vi "20210415_00_ATA_FPGA.vi"() -> ()   [LabVIEW 2018]
doc: "This FPGA VI transfers data samples to the host using a stream. The stream is controlled from the host."
uses:
  <vilib>/Platform/TimedLoop/XDataNode/wakeup.ctl
  <vilib>/Platform/TimedLoop/XDataNode/XDNodeRunTimeDep.lvlib
  <vilib>/Platform/TimedLoop/XDataNode/nitl_modes.ctl
  <vilib>/Platform/TimedLoop/XDataNode/timing_clust.ctl
  <vilib>/Platform/TimedLoop/XDataNode/XDataNode.xnode
  <vilib>/eio/EIONode/EIONode.xnode
  <vilib>/rvi/eio/common/nirviEmuTemplateMethod_errors.vi
  <vilib>/rvi/DataTransferAndStorage/Container/XNode/niFpgaContainer.xnode
  <instrlib>/_niInstr/Basic Elements/v1/FPGA/niInstr Basic Elements v1 FPGA.lvlib
  <vilib>/rvi/FXPMathLib/FxpInterpret/XNode/nifxpmath_Interpret.xnode
  <vilib>/rvi/FXPMathLib/FxpMul/XNode/nifxpmath_Multiplier.xnode
  <vilib>/rvi/FXPMathLib/sim/FxpSim.dll
  <vilib>/rvi/FXPMathLib/FxpAdd/XNode/nifxpmath_Add.xnode
  <vilib>/rvi/Analysis/measure/FFT/XNode/niFpgaFFT.xnode
  <instrlib>/_niInstr/Basic Elements/v1/FPGA/Private/Count Up U32.vi
  <vilib>/rvi/Memory/Memory_Emulation/niFpgaMemoryEmulationRefIn.vi
  <vilib>/fxp/LVFixedPointQuantizationPolicyTypeDef.ctl
  <vilib>/rvi/Analysis/measure/FFT/simModelSupport/niFpgaFFTSimDfxp.ctl
  <vilib>/rvi/Analysis/measure/FFT/simModelSupport/niFpgaFFTSimArithmeticProperties.ctl
  <vilib>/rvi/Analysis/measure/FFT/simModelSupport/niFPGA FFT Sim Types.ctl
  <vilib>/rvi/Analysis/measure/FFT/simModelSupport/niFPGA FFT Outside SCTL Sim Properties.ctl
  <vilib>/rvi/Analysis/measure/FFT/simModelSupport/niFpgaFFTSimModelOutsideSCTLCore.vi
  <vilib>/rvi/LocalResourceManager/LocalResourceManager.xnode
  <vilib>/rvi/DataTransferAndStorage/Container/Common/niFpgaContainerGetUniqueNameForEmu.vi
  <vilib>/rvi/DataTransferAndStorage/Container/Common/niFpgaContainerSetEmuInfo.vi
  <vilib>/rvi/eio/common/nirviEmuReportErrorAndStop.vi
  <vilib>/rvi/FIFO/Fifo_Resource/niFpgaFifoEmulationRefIn.vi
  <vilib>/rvi/FIFO/Fifo_Resource/nirvififoEmulationRead.vi
  <vilib>/rvi/interface/RandomDataEmulation/nirviRandomDataFpgaMultiElementTemplate.vi
  <instrlib>/_niInstr/Basic Elements/v1/FPGA/Private/Count Up U16.vi
  FPGA_Controls/FilterStageEnum.ctl
  FPGA_Controls/FPGA_Enable_Clust.ctl
  FPGA_Controls/FPGA_Shift_Enable.ctl
  <instrlib>/_niInstr/Basic Elements/v1/FPGA/Private/Count Up U8.vi
  FPGA_Controls/FPGA_Scale_Clust.ctl
  FPGA_Controls/FPGA_Probe_Clust.ctl
panel:
  out "Write to FIFO 2":bool
  out "Write to FIFO":bool
  in  "EnableFIFO":bool
  out "AI0_Unshifted_Index":u32
  out "AI0_Co_Beac_Q_Index":fxp<+/-,24,1>
  out "AI0_Co_I_Index":fxp<+/-,24,1>
  out "MaxMeas":fxp<+/-,24,1>
  in  "Ramp?":bool
  out "AI1_Over":bool
  out "AI0_Over":bool
  in  "Simulate?":bool
  out "Chan1_Beac_QProbe":T1
  out "Chan1_Beac_IProbe":T1
  out "Chan1_Cal_QProbe":T1
  out "Chan0_Beac_QProbe":T1
  out "Chan0_Beac_IProbe":T1
  out "Chan0_Cal_QProbe":T1
  out "NoiseFloorFFT_LoopCount 2":i32
  out "ReceiverTimed Out 2":bool
  out "SuccessiveIndeces 2":u16[](array[numeric])
  in  "#Avg 2":u16=1
  in  "ScaleMeasurement 2":fxp<+/-,16,1>
  in  "Scale_Step1_2":fxp<+/-,17,17>
  in  "EnableStep1_2":bool
  out "Probe 2_2":fxp<+/-,16,16>
  out "Probe 3_2":fxp<+/-,16,1>
  out "Probe 5_2":fxp<+/-,16,2>
  out "Probe 7_2":fxp<+/-,18,1>
  in  "Scale_NoiseFloor 2":fxp<+/-,30,30>
  out "Probe 21_2":fxp<+/-,24,5>
  out "Probe 22_2":fxp<+/-,54,35>
  out "Probe 23_2":fxp<+/-,54,1>
  out "Probe 24_2":fxp<+/-,16,1>
  in  "Offset 2":fxp<+/-,16,16>
  in  "Scale 2":T2={"Scale_Step4"=1.0, "Scale_Step5"=1.0, "Scale_Step6"=1.0, "Scale_Step7"=1.0}
  in  "Enable 2":T3
  in  "FreqShiftCal 2":fxp<+/-,48,0> format="%#.48g"
  out "Chan1_Cal_IProbe":T1
  in  "FreqShiftBeac 2":fxp<+/-,48,0> format="%#.48g"
  out "NoiseFloorFIFOTimeOut 2":bool
  out "Sends 2":u32
  in  "SampleCountReset 2":u32=125000000
  out "Probe 1_2":i16
  out "Probe Offsetd 2":fxp<+/-,16,16>
  out "Probe Offsetd":fxp<+/-,16,16>
  in  "Sample Clock Commit":bool
  in  "Sample Clock Select":u8
  out "SPI Idle":bool
  out "Configuration Error":bool
  out "Synthesizer Locked":bool
  out "Probe 1":i16
  in  "#Avg":u16=1
  in  "SampleCountReset":u32=125000000
  out "ReceiverTimed Out":bool
  out "Sends":u32
  out "SuccessiveIndeces":u16[](array[numeric])
  out "NoiseFloorFFT_LoopCount":i32
  out "NoiseFloorFIFOTimeOut":bool
  in  "FreqShiftBeac":fxp<+/-,48,0> format="%#.48g"
  out "AI0_Cal_IProbe":T1
  in  "Scale":T2={"Scale_Step4"=1.0, "Scale_Step5"=1.0, "Scale_Step6"=1.0, "Scale_Step7"=1.0}
  in  "Enable":T3
  in  "Offset":fxp<+/-,16,16>
  out "Probe 24":fxp<+/-,16,1>
  out "Probe 23":fxp<+/-,54,1>
  out "Probe 22":fxp<+/-,54,35>
  out "Probe 21":fxp<+/-,24,5>
  in  "Scale_NoiseFloor":fxp<+/-,30,30>
  out "Probe 7":fxp<+/-,18,1>
  out "Probe 5":fxp<+/-,16,2>
  out "Probe 3":fxp<+/-,16,1>
  out "Probe 2":fxp<+/-,16,16>
  in  "EnableStep1":bool
  in  "Scale_Step1":fxp<+/-,17,17>
  in  "ScaleMeasurement":fxp<+/-,16,1>
  in  "FreqShiftCal":fxp<+/-,48,0> format="%#.48g"
  out "IO Module\\Initialization Done":bool
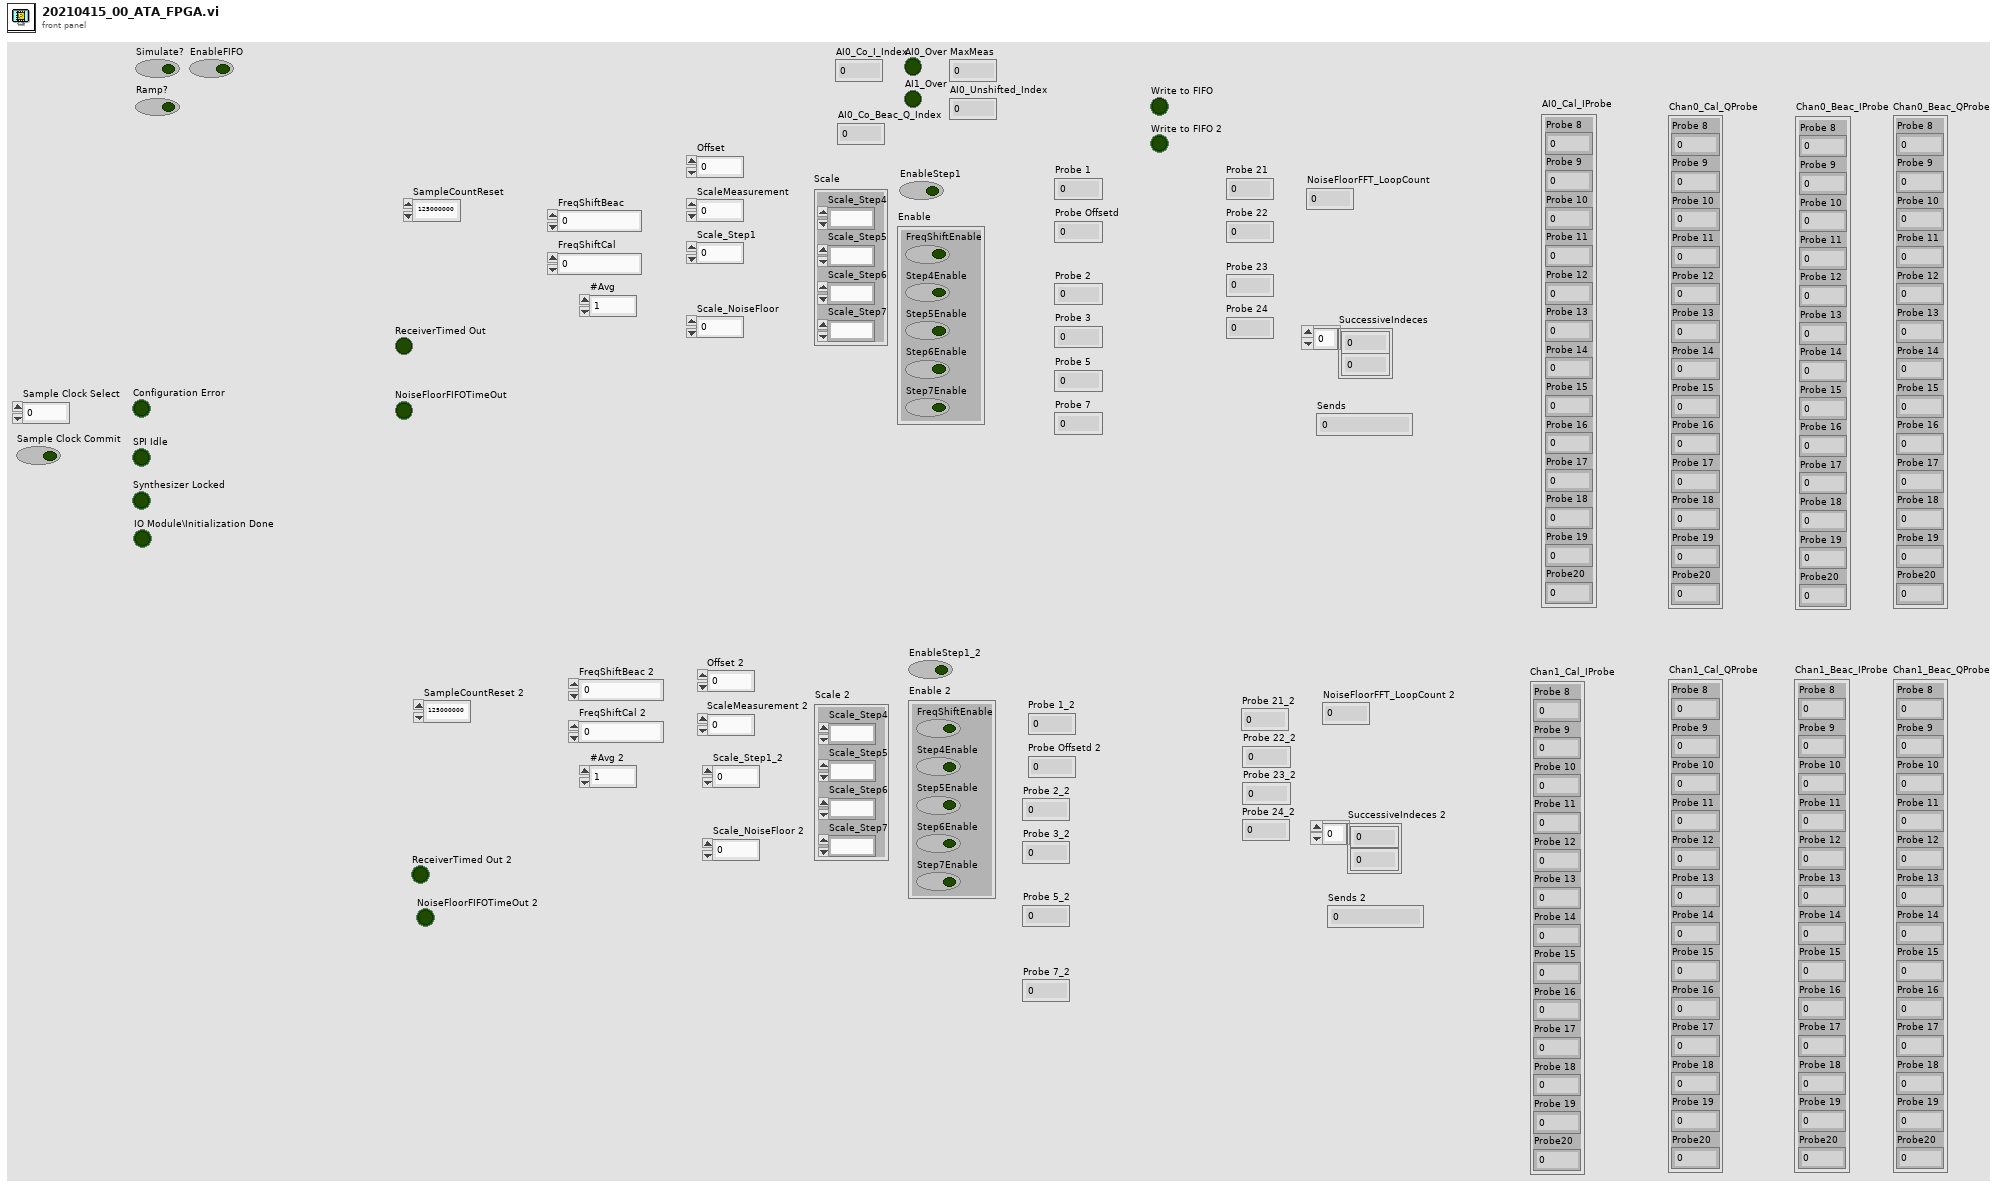
[diagram p1: front panel]
types:
  T1 = typedef "FPGA_Probe_Clust.ctl" = cluster{"Probe 8":fxp<+/-,18,1>, "Probe 9":fxp<+/-,24,1>, "Probe 10":fxp<+/-,24,1>, "Probe 11":fxp<+/-,24,1>, "Probe 12":fxp<+/-,47,24>, "Probe 13":fxp<+/-,24,1>, "Probe 14":fxp<+/-,25,2>, "Probe 15":fxp<+/-,48,25>, "Probe 16":fxp<+/-,24,1>, "Probe 17":fxp<+/-,25,2>, "Probe 18":fxp<+/-,48,25>, "Probe 19":fxp<+/-,24,1>, "Probe20":fxp<+/-,24,1>}
  T2 = typedef "FPGA_Scale_Clust.ctl" = cluster{"Scale_Step4":fxp<+/-,23,23>, "Scale_Step5":fxp<+/-,23,23>, "Scale_Step6":fxp<+/-,23,23>, "Scale_Step7":fxp<+/-,23,23>}
  T3 = typedef "FPGA_Enable_Clust.ctl" = cluster{"FreqShiftEnable":bool, "Step4Enable":bool, "Step5Enable":bool, "Step6Enable":bool, "Step7Enable":bool}
  T4 = typedef "XDNodeRunTimeDep.lvlib/timing_clust.ctl" = cluster{"Expected End [f-1]":u64, "Actual End [f-1]":u64, "Finished Late? [f-1]":bool, "Expected End [i-1]":u64, "Actual End [i-1]":u64, "Finished Late? [i-1]":bool, "Expected Start [i]":u64, "Actual Start [i]":u64, "Expected Start [f]":u64, "Actual Start [f]":u64, "Source Name":string, "Structure Name":string, "Period":i64, "Deadline":i64, "Offset":i64, "Start":i64, "Priority":i32, "Timeout":i32, "Mode":T5, "Wakeup Reason":T6, "Error":errorcluster, "Source Type":string, "Secondary Source Type":string, "Global End Time":u64, "Global Start Time":u64, "Frame Duration":u64, "Iteration Duration":u64, "Assigned CPU":i32, "I/O Scan Engine Mode":u32}
  T5 = typedef "XDNodeRunTimeDep.lvlib/nitl_modes.ctl" = enum32{"No Change", "Process missed periods, maintain original phase", "Discard missed periods, maintain original phase", "Process missed periods, ignore original phase", "Discard missed periods, ignore original phase"}
  T6 = typedef "XDNodeRunTimeDep.lvlib/wakeup.ctl" = enum32{"Normal", "Aborted", "Asynchronous wakeup", "Timing source error", "Timed loop error", "Timeout"}
  T7 = typedef "FPGA_Shift_Enable.ctl" = cluster{"EnableFIFO":bool, "EnableStages":T3}
  T8 = typedef "FilterStageEnum.ctl" = enum16{"Digitiz0", "Digitiz1", "ScaleMeas", "Scale1", "Scale4", "Scale5", "Scale6", "Scale7"}
  T9 = typedef "FPGA_ShiftOutput.ctl" = cluster{"Index":fxp<+/-,24,1>, "output valid":bool, "Data out":fxp<+/-,24,1>, "Probe":T1}
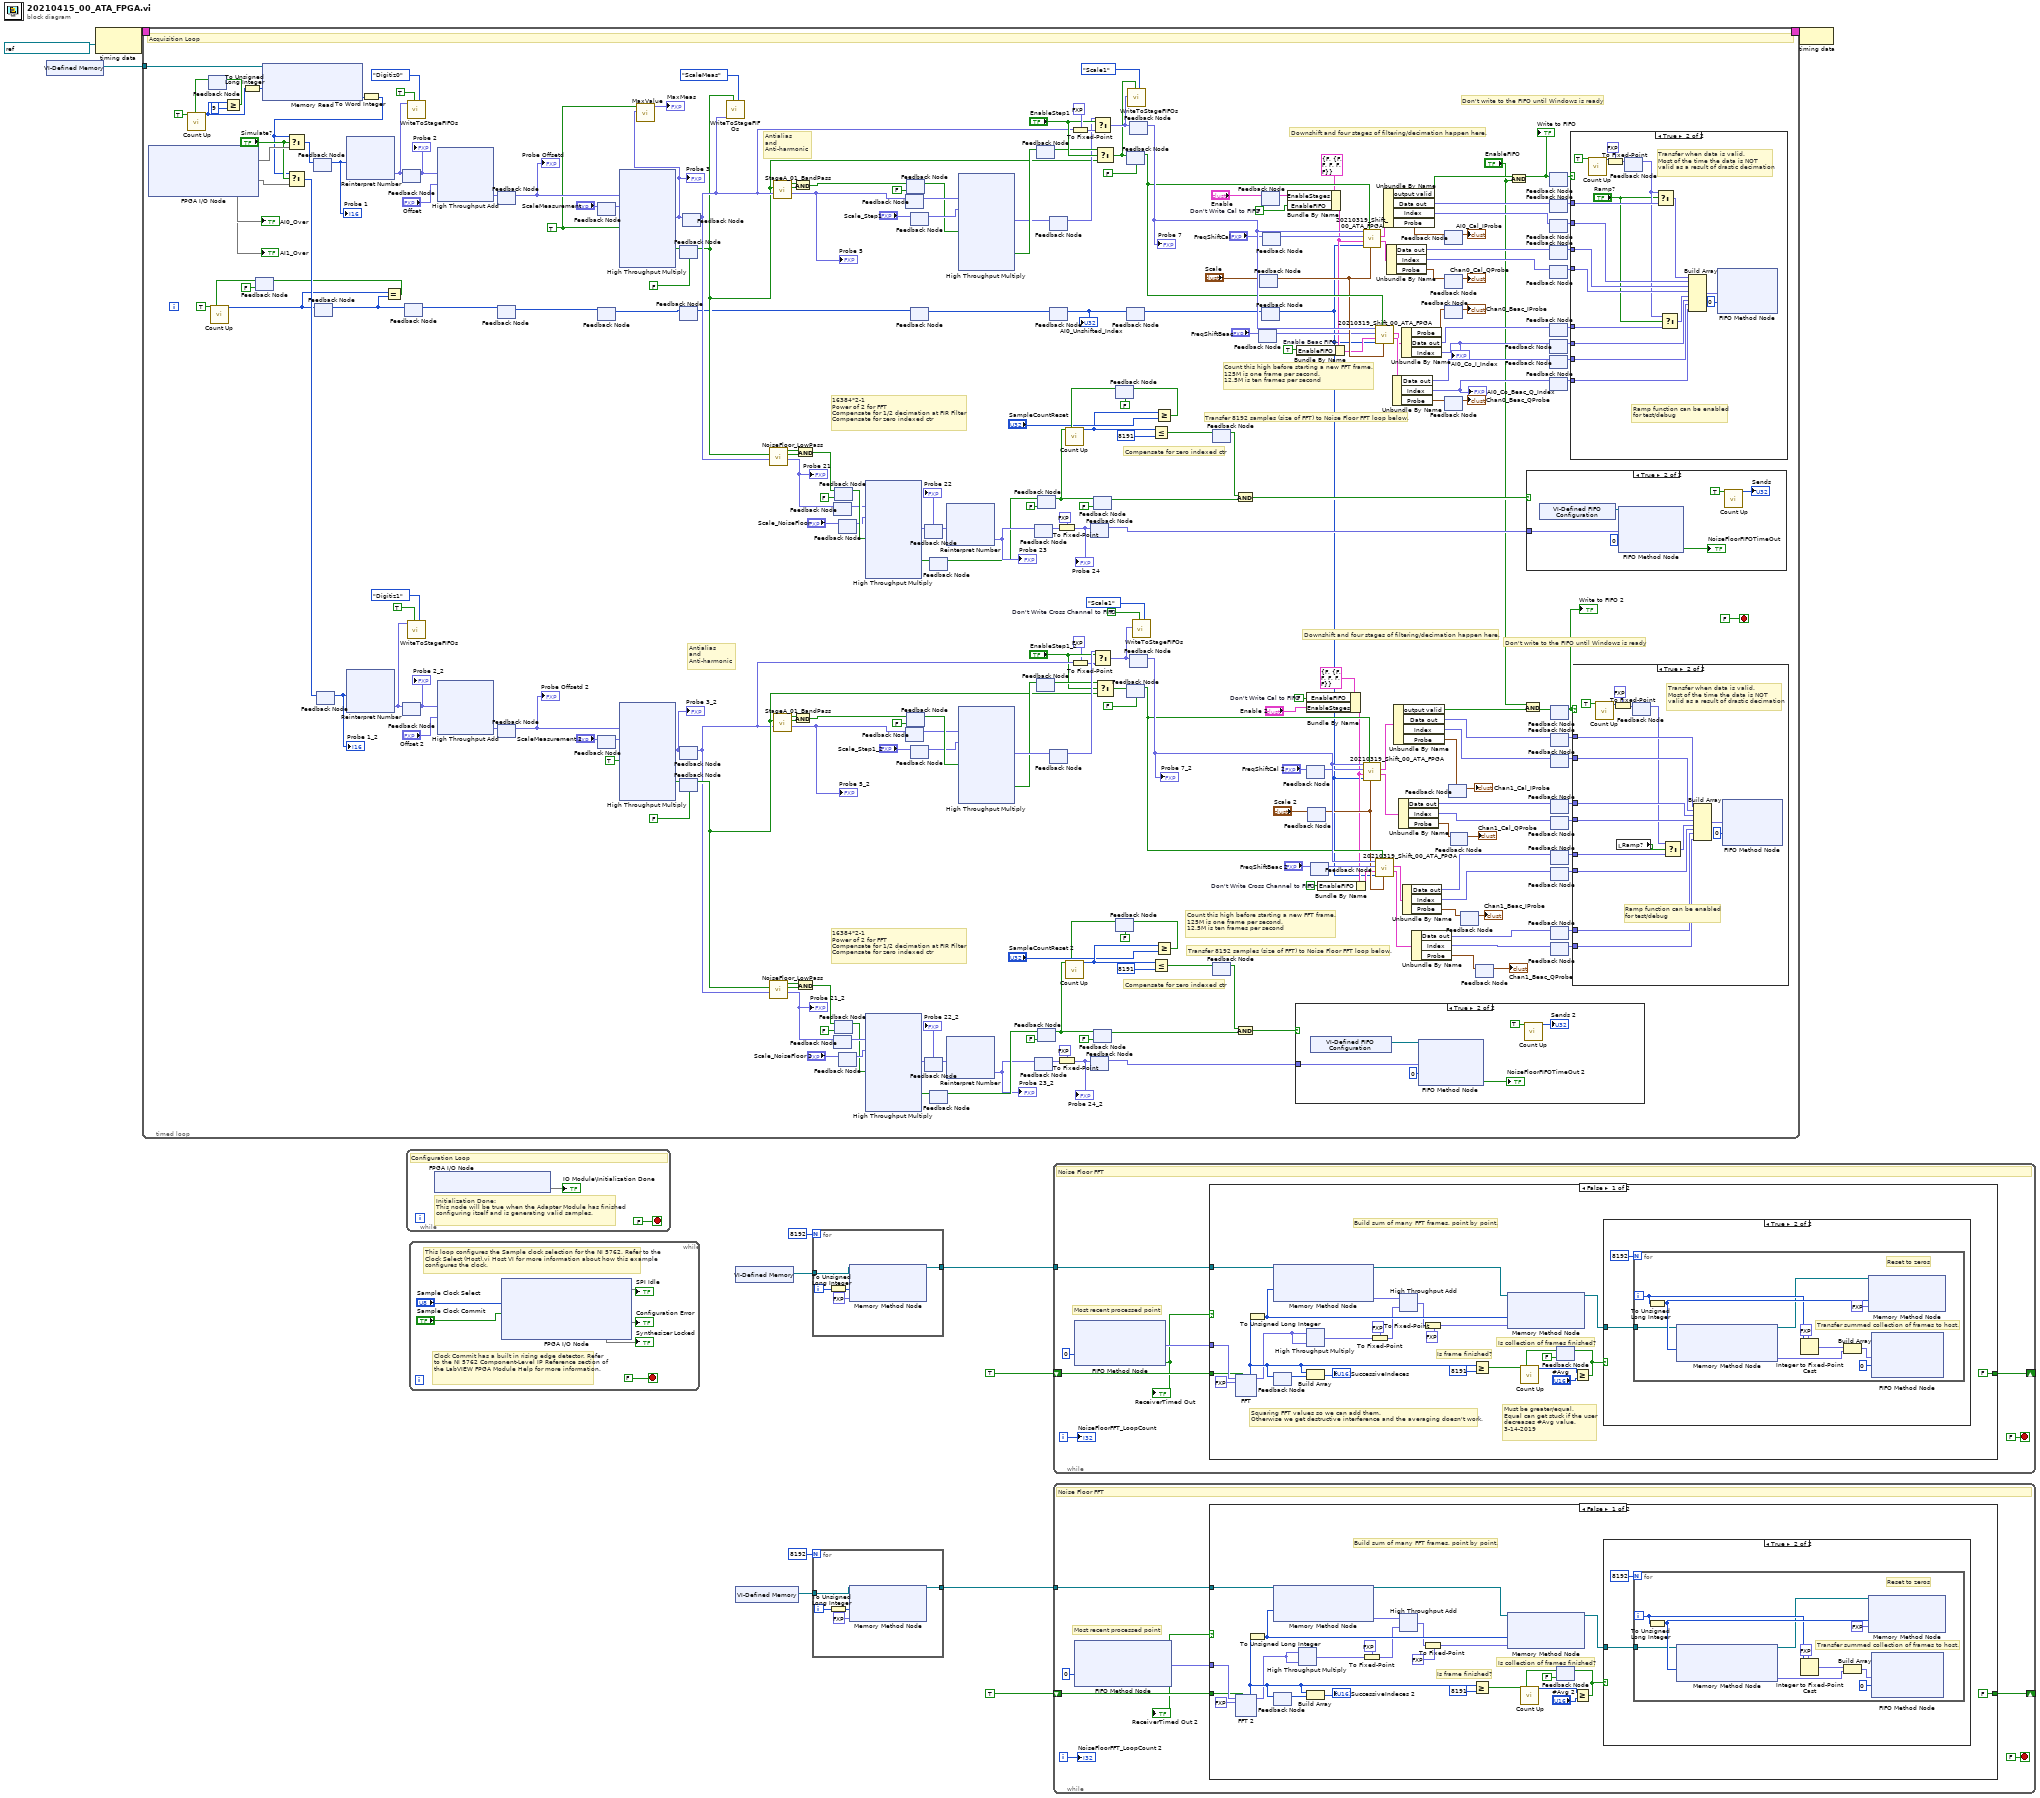
[diagram p0: block diagram]
diagram:
  n1 = xnode "VI-Defined Memory"() -> ("Memory Out"=w1:refnum<k21>)
  n2 = node-c288(refnum<k21> "IO Module\\Data Clock" ("Source Name")) -> (w12:T4)
  n3 = timed-loop {
    timing: w12 -> [_]
    timing-out: [_] -> w11
    tunnel: w1 -> [w111]
    stop <- FALSE stop-if-true
    w59 = FALSE  # Don't Write Cal to FIFO
    w56 = TRUE  # Enable Beac FIFO
    w87 = FALSE  # Don't Write Cross Channel to FIFO
    w45 = FALSE  # Don't Write Cross Channel to FIFO
    w51 = FALSE  # Don't Write Cal to FIFO
    w100 = TRUE ("input valid")
    # "Don't write to the FIFO until Windows is ready"
    # "Don't write to the FIFO until Windows is ready"
    # "Downshift and four stages of filtering/decimation happen here."
    # "Downshift and four stages of filtering/decimation happen here."
    # "Antialias\nand\nAnti-harmonic"
    # "Compensate for zero indexed ctr"
    # "16384*2-1\nPower of 2 for FFT\nCompensate for 1/2 decimation at FIR Filter\nCompensate for zero indexed ctr"
    # "Transfer 8192 samples (size of FFT) to Noise Floor FFT loop below."
    # "Count this high before starting a new FFT frame.\n125M is one frame per second.\n12.5M is ten frames per second"
    # "Antialias\nand\nAnti-harmonic"
    # "Compensate for zero indexed ctr"
    # "16384*2-1\nPower of 2 for FFT\nCompensate for 1/2 decimation at FIR Filter\nCompensate for zero indexed ctr"
    # "Transfer 8192 samples (size of FFT) to Noise Floor FFT loop below."
    # "Count this high before starting a new FFT frame.\n125M is one frame per second.\n12.5M is ten frames per second"
    # "Acquisition Loop"
    n4 = xnode "FPGA I/O Node"() -> ("IO Module\\AI 0 Data"=w110, "IO Module\\AI 0 Over Range"=→"AI0_Over", "IO Module\\AI 1 Data"=w105, "IO Module\\AI 1 Over Range"=→"AI1_Over")  [unwired: 4 in, 4 out]
    n5 = feedback #1() -> (w112:bool)  [unwired: 1 in]
    n6 = call-poly <instrlib>:"Count Up.vi"("increment"=TRUE, "reset"=w112) -> ("count out"=w115:u8)  [unwired: 13 in]
    n7 = Greater Or Equal?(x=w115, y=u8 9) -> (x >= y?=w113:bool)
    n8 = feedback-in #1(w113) -> ()
    n9 = To Unsigned Long Integer(number=w115) -> (unsigned 32bit integer=w117:u32)
    n10 = feedback #2(FALSE) -> (w21:bool)
    n11 = call-poly <instrlib>:"Count Up.vi"("increment"=TRUE, "reset"=w21) -> ("count out"=w19:u32)  [unwired: 13 in]
    n12 = xnode ("Memory Read")("Address"=w117, "Memory In"=w111) -> ("Data"=w108:i8)  [unwired: 1 out]
    n13 = feedback #3() -> (w219:i16)  [unwired: 1 in]
    "Probe 1" <- w219
    n14 = feedback #4() -> (w18:u32)  [unwired: 1 in]
    n15 = feedback-in #4(w19) -> ()
    n16 = feedback #5() -> (w200:i16)  [unwired: 1 in]
    "Probe 1_2" <- w200
    n17 = xnode "Reinterpret Number"("x"=w219) -> ("y"=w91:fxp<+/-,16,16>)
    n18 = xnode "Reinterpret Number"("x"=w200) -> ("y"=w90:fxp<+/-,16,16>)
    n19 = To Word Integer(number=w108) -> (16bit integer=w104:i16)
    n20 = Select(t=w104, s="Simulate?", f=w110) -> (s? t:f=w109:i16)
    n21 = Select(t=w104, s="Simulate?", f=w105) -> (s? t:f=w106:i16)
    n22 = feedback-in #3(w109) -> ()
    n23 = feedback-in #5(w106) -> ()
    n24 = Equal?(x=w19, y=w18) -> (x = y?=w22:bool)
    n25 = feedback-in #2(w22) -> ()
    n26 = feedback #6() -> (w232:fxp<+/-,16,16>)  [unwired: 1 in]
    "Probe 2" <- w232
    n27 = feedback-in #6(w91) -> ()
    n28 = feedback #7() -> (w191:fxp<+/-,16,16>)  [unwired: 1 in]
    "Probe 2_2" <- w191
    n29 = feedback-in #7(w90) -> ()
    n30 = feedback #8() -> (w23:u32)  [unwired: 1 in]
    n31 = feedback-in #8(w18) -> ()
    n32 = call "WriteToStageFIFOs.vi"("Stage"=FilterStageEnum."Digitiz0", "Enable"=TRUE, "Digitiz"=w91) -> ()  [unwired: 9 in]
    n33 = call "WriteToStageFIFOs.vi"("Stage"=FilterStageEnum."Digitiz1", "Enable"=TRUE, "Digitiz"=w90) -> ()  [unwired: 9 in]
    n34 = xnode ("High Throughput Add")("x"=w232, "y"="Offset") -> ("x+y"=w231:fxp<+/-,16,16>)
    n35 = xnode ("High Throughput Add")("x"=w191, "y"="Offset 2") -> ("x+y"=w93:fxp<+/-,16,16>)
    n36 = feedback #9() -> (w101:fxp<+/-,16,16>)  [unwired: 1 in]
    "Probe Offsetd" <- w101
    n37 = feedback-in #9(w231) -> ()
    n38 = feedback #10() -> (w80:u32)  [unwired: 1 in]
    n39 = feedback-in #10(w23) -> ()
    n40 = feedback #11() -> (w92:fxp<+/-,16,16>)  [unwired: 1 in]
    "Probe Offsetd 2" <- w92
    n41 = feedback-in #11(w93) -> ()
    n42 = feedback #12() -> (w260:fxp<+/-,16,1>)  [unwired: 1 in]
    n43 = feedback-in #12("ScaleMeasurement") -> ()
    n44 = feedback #13() -> (w79:u32)  [unwired: 1 in]
    n45 = feedback-in #13(w80) -> ()
    n46 = feedback #14() -> (w161:fxp<+/-,16,1>)  [unwired: 1 in]
    n47 = feedback-in #14("ScaleMeasurement 2") -> ()
    n48 = xnode ("High Throughput Multiply")("x"=w101, "y"=w260, "input valid"=w100) -> ("x*y"=w99:fxp<+/-,16,1>, "output valid"=w234:bool)  [unwired: 1 in, 1 out]
    "Probe 3" <- w99
    n49 = xnode ("High Throughput Multiply")("x"=w92, "y"=w161, "input valid"=TRUE) -> ("x*y"=w158:fxp<+/-,16,1>, "output valid"=w189:bool)  [unwired: 1 in, 1 out]
    "Probe 3_2" <- w158
    n50 = call "MaxValue.vi"("NewValue"=w99, "DataValid"=w100) -> ("Max"=→"MaxMeas":fxp<+/-,24,1>)  [unwired: 9 in]
    n51 = feedback #15(FALSE ("output valid")) -> (w82:bool)
    n52 = feedback-in #15(w234) -> ()
    n53 = feedback #16() -> (w78:u32)  [unwired: 1 in]
    n54 = feedback-in #16(w79) -> ()
    n55 = feedback #17() -> (w203:fxp<+/-,16,1>)  [unwired: 1 in]
    n56 = feedback-in #17(w158) -> ()
    n57 = feedback #18(FALSE ("output valid")) -> (w205:bool)
    n58 = feedback-in #18(w189) -> ()
    n59 = feedback #19() -> (w83:fxp<+/-,16,1>)  [unwired: 1 in]
    n60 = feedback-in #19(w99) -> ()
    n61 = call "WriteToStageFIFOs.vi"("Stage"=FilterStageEnum."ScaleMeas", "Enable"=w82, "ScaleMeas"=w83) -> ()  [unwired: 9 in]
    n62 = call "NoiseFloor_LowPass.vi"("s_axis_data_tdata"=w83, "s_axis_data_tvalid"=w82) -> ("m_axis_data_tdata"=w244:fxp<+/-,24,5>, "m_axis_data_tvalid"=w251:bool, "s_axis_data_tready"=w252:bool)  [unwired: 7 in]
    "Probe 21" <- w244
    n63 = call "NoiseFloor_LowPass.vi"("s_axis_data_tdata"=w203, "s_axis_data_tvalid"=w205) -> ("m_axis_data_tdata"=w179:fxp<+/-,24,5>, "m_axis_data_tvalid"=w172:bool, "s_axis_data_tready"=w171:bool)  [unwired: 7 in]
    "Probe 21_2" <- w179
    n64 = call "StageA_01_BandPass.vi"("s_axis_data_tdata"=w83, "s_axis_data_tvalid"=w82) -> ("m_axis_data_tdata"=w216:fxp<+/-,16,2>, "m_axis_data_tvalid"=w265:bool, "s_axis_data_tready"=w266:bool)  [unwired: 7 in]
    "Probe 5" <- w216
    n65 = call "StageA_01_BandPass.vi"("s_axis_data_tdata"=w203, "s_axis_data_tvalid"=w205) -> ("m_axis_data_tdata"=w204:fxp<+/-,16,2>, "m_axis_data_tvalid"=w155:bool, "s_axis_data_tready"=w154:bool)  [unwired: 7 in]
    "Probe 5_2" <- w204
    n66 = And(x=w266, y=w265) -> (x .and. y?=w217:bool)
    n67 = And(x=w154, y=w155) -> (x .and. y?=w202:bool)
    n68 = And(x=w252, y=w251) -> (x .and. y?=w243:bool)
    n69 = And(x=w171, y=w172) -> (x .and. y?=w180:bool)
    n70 = feedback #20() -> (w245:fxp<+/-,24,5>)  [unwired: 1 in]
    n71 = feedback-in #20(w244) -> ()
    n72 = feedback #21() -> (w178:fxp<+/-,24,5>)  [unwired: 1 in]
    n73 = feedback-in #21(w179) -> ()
    n74 = feedback #22(FALSE ("s_axis_data_tvalid")) -> (w248:bool)
    n75 = feedback-in #22(w243) -> ()
    n76 = feedback #23(FALSE ("s_axis_data_tvalid")) -> (w175:bool)
    n77 = feedback-in #23(w180) -> ()
    n78 = feedback #24() -> (w247:fxp<+/-,30,30>)  [unwired: 1 in]
    n79 = feedback-in #24("Scale_NoiseFloor") -> ()
    n80 = feedback #25() -> (w176:fxp<+/-,30,30>)  [unwired: 1 in]
    n81 = feedback-in #25("Scale_NoiseFloor 2") -> ()
    n82 = xnode ("High Throughput Multiply")("x"=w245, "y"=w247, "input valid"=w248) -> ("x*y"=w240:fxp<+/-,54,35>, "output valid"=w237:bool)  [unwired: 1 in, 1 out]
    "Probe 22" <- w240
    n83 = xnode ("High Throughput Multiply")("x"=w178, "y"=w176, "input valid"=w175) -> ("x*y"=w183:fxp<+/-,54,35>, "output valid"=w186:bool)  [unwired: 1 in, 1 out]
    "Probe 22_2" <- w183
    n84 = feedback #26() -> (w262:fxp<+/-,16,2>)  [unwired: 1 in]
    n85 = feedback-in #26(w216) -> ()
    n86 = feedback #27() -> (w159:fxp<+/-,16,2>)  [unwired: 1 in]
    n87 = feedback-in #27(w204) -> ()
    n88 = feedback #28(FALSE ("s_axis_data_tvalid")) -> (w258:bool)
    n89 = feedback-in #28(w217) -> ()
    n90 = feedback #29(FALSE ("s_axis_data_tvalid")) -> (w163:bool)
    n91 = feedback-in #29(w202) -> ()
    n92 = feedback #30() -> (w259:fxp<+/-,17,17>)  [unwired: 1 in]
    n93 = feedback-in #30("Scale_Step1") -> ()
    n94 = feedback #31() -> (w77:u32)  [unwired: 1 in]
    n95 = feedback-in #31(w78) -> ()
    n96 = feedback #32() -> (w162:fxp<+/-,17,17>)  [unwired: 1 in]
    n97 = feedback-in #32("Scale_Step1_2") -> ()
    n98 = feedback #33() -> (w239:fxp<+/-,54,35>)  [unwired: 1 in]
    n99 = feedback-in #33(w240) -> ()
    n100 = feedback #34() -> (w184:fxp<+/-,54,35>)  [unwired: 1 in]
    n101 = feedback-in #34(w183) -> ()
    n102 = feedback #35() -> (w236:bool)  [unwired: 1 in]
    n103 = feedback-in #35(w237) -> ()
    n104 = feedback #36() -> (w187:bool)  [unwired: 1 in]
    n105 = feedback-in #36(w186) -> ()
    n106 = xnode "Reinterpret Number"("x"=w239) -> ("y"=w238:fxp<+/-,54,1>)
    "Probe 23" <- w238
    n107 = xnode "Reinterpret Number"("x"=w184) -> ("y"=w185:fxp<+/-,54,1>)
    "Probe 23_2" <- w185
    n108 = xnode ("High Throughput Multiply")("x"=w262, "y"=w259, "input valid"=w258) -> ("x*y"=w213:fxp<+/-,18,1>, "output valid"=w215:bool)  [unwired: 1 in, 1 out]
    n109 = xnode ("High Throughput Multiply")("x"=w159, "y"=w162, "input valid"=w163) -> ("x*y"=w208:fxp<+/-,18,1>, "output valid"=w206:bool)  [unwired: 1 in, 1 out]
    n110 = feedback #37() -> (w241:fxp<+/-,54,1>)  [unwired: 1 in]
    n111 = feedback-in #37(w238) -> ()
    n112 = feedback #38() -> (w182:fxp<+/-,54,1>)  [unwired: 1 in]
    n113 = feedback-in #38(w185) -> ()
    n114 = feedback #39() -> (w214:bool)  [unwired: 1 in]
    n115 = feedback-in #39(w215) -> ()
    n116 = feedback #40() -> (w207:bool)  [unwired: 1 in]
    n117 = feedback-in #40(w206) -> ()
    n118 = feedback #41(FALSE ("output valid")) -> (w230:bool)
    n119 = feedback-in #41(w236) -> ()
    n120 = feedback #42(FALSE ("output valid")) -> (w192:bool)
    n121 = feedback-in #42(w187) -> ()
    n122 = feedback #43() -> (w212:fxp<+/-,18,1>)  [unwired: 1 in]
    n123 = feedback-in #43(w213) -> ()
    n124 = feedback #44() -> (w76:u32)  [unwired: 1 in]
    "AI0_Unshifted_Index" <- w76
    n125 = feedback-in #44(w77) -> ()
    n126 = feedback #45() -> (w209:fxp<+/-,18,1>)  [unwired: 1 in]
    n127 = feedback-in #45(w208) -> ()
    n128 = To Fixed-Point(fixed-point type=fxp<+/-,16,1> 0.0, number=w241) -> (fixed-point=w220:fxp<+/-,16,1>)
    "Probe 24" <- w220
    n129 = To Fixed-Point(fixed-point type=fxp<+/-,16,1> 0.0, number=w182) -> (fixed-point=w199:fxp<+/-,16,1>)
    "Probe 24_2" <- w199
    n130 = To Fixed-Point(fixed-point type=fxp<+/-,18,1> 0.0, number=w83) -> (fixed-point=w256:fxp<+/-,18,1>)
    n131 = To Fixed-Point(fixed-point type=fxp<+/-,18,1> 0.0, number=w203) -> (fixed-point=w166:fxp<+/-,18,1>)
    n132 = feedback #46() -> (w221:fxp<+/-,16,1>)  [unwired: 1 in]
    n133 = feedback-in #46(w220) -> ()
    n134 = feedback #47() -> (w198:fxp<+/-,16,1>)  [unwired: 1 in]
    n135 = feedback-in #47(w199) -> ()
    n136 = feedback #48(FALSE ("output valid")) -> (w228:bool)
    n137 = feedback-in #48(w230) -> ()
    n138 = feedback #49(FALSE ("output valid")) -> (w194:bool)
    n139 = feedback-in #49(w192) -> ()
    n140 = Select(t=w212, s="EnableStep1", f=w256) -> (s? t:f=w95:fxp<+/-,18,1>)
    n141 = Select(t=w209, s="EnableStep1_2", f=w166) -> (s? t:f=w88:fxp<+/-,18,1>)
    n142 = Select(t=w214, s="EnableStep1", f=w82) -> (s? t:f=w81:bool)
    n143 = Select(t=w207, s="EnableStep1_2", f=w205) -> (s? t:f=w164:bool)
    n144 = feedback #50(FALSE ("reset")) -> (w271:bool)
    n145 = call-poly <instrlib>:"Count Up.vi"("increment"=w230, "reset"=w271) -> ("count out"=w264:u32)  [unwired: 13 in]
    n146 = feedback #51(FALSE ("reset")) -> (w149:bool)
    n147 = call-poly <instrlib>:"Count Up.vi"("increment"=w192, "reset"=w149) -> ("count out"=w156:u32)  [unwired: 13 in]
    n148 = feedback #52(FALSE ("s_axis_data_tvalid")) -> (w147:bool)
    n149 = feedback-in #52(w81) -> ()
    n150 = feedback #53() -> (w75:u32)  [unwired: 1 in]
    n151 = feedback-in #53(w76) -> ()
    n152 = feedback #54(FALSE ("s_axis_data_tvalid")) -> (w141:bool)
    n153 = feedback-in #54(w164) -> ()
    n154 = call "WriteToStageFIFOs.vi"("Stage"=FilterStageEnum."Scale1", "Enable"=w81, "Scale1"=w95) -> ()  [unwired: 9 in]
    n155 = feedback #55() -> (w211:fxp<+/-,18,1>)  [unwired: 1 in]
    "Probe 7" <- w211
    n156 = feedback-in #55(w95) -> ()
    n157 = feedback #56() -> (w210:fxp<+/-,18,1>)  [unwired: 1 in]
    "Probe 7_2" <- w210
    n158 = feedback-in #56(w88) -> ()
    n159 = call "WriteToStageFIFOs.vi"("Stage"=FilterStageEnum."Scale1", "Enable"=w87, "Scale1"=w88) -> ()  [unwired: 9 in]
    n160 = Less Or Equal?(x=w264, y=u32 8191) -> (x <= y?=w272:bool)
    n161 = Less Or Equal?(x=w156, y=u32 8191) -> (x <= y?=w148:bool)
    n162 = Greater Or Equal?(x=w264, y="SampleCountReset") -> (x >= y?=w268:bool)
    n163 = feedback-in #50(w268) -> ()
    n164 = Greater Or Equal?(x=w156, y="SampleCountReset 2") -> (x >= y?=w152:bool)
    n165 = feedback-in #51(w152) -> ()
    n166 = feedback #57() -> (w229:bool)  [unwired: 1 in]
    n167 = feedback-in #57(w272) -> ()
    n168 = feedback #58() -> (w193:bool)  [unwired: 1 in]
    n169 = feedback-in #58(w148) -> ()
    n170 = And(x=w229, y=w228) -> (x .and. y?=w227:bool)
    n171 = And(x=w193, y=w194) -> (x .and. y?=w195:bool)
    n172 = feedback #59() -> (w130:fxp<+/-,48,0>)  [unwired: 1 in]
    n173 = feedback-in #59("FreqShiftBeac") -> ()
    n174 = feedback #60() -> (w132:T2)  [unwired: 1 in]
    n175 = feedback-in #60("Scale") -> ()
    n176 = feedback #61() -> (w60:T3)  [unwired: 1 in]
    n177 = feedback-in #61("Enable") -> ()
    n178 = feedback #62() -> (w17:u32)  [unwired: 1 in]
    n179 = feedback-in #62(w75) -> ()
    n180 = feedback #63() -> (w128:fxp<+/-,48,0>)  [unwired: 1 in]
    n181 = feedback-in #63("FreqShiftCal") -> ()
    n182 = Bundle By Name(cluster=T7 {"EnableFIFO"=FALSE, "EnableStages"={"FreqShiftEnable"=FALSE, "Step4Enable"=FALSE, "Step5Enable"=FALSE, "Step6Enable"=FALSE, "Step7Enable"=FALSE}}, "EnableStages"=w60, "EnableFIFO"=w59) -> (w58:T7)
    n183 = case shown="True" w195 {
      tunnel: w198 -> [_ w278]
      frame False {
      }
      frame True {
        n184 = xnode "VI-Defined FIFO Configuration"() -> ("FIFO Out"=w273:refnum<k21>)
        n185 = xnode ("FIFO Method Node")("Element"=w278, "Timeout"=0, "FIFO In"=w273) -> ("Timed Out?"=→"NoiseFloorFIFOTimeOut 2":bool)  [unwired: 1 out]
        n186 = call-poly <instrlib>:"Count Up.vi"("increment"=TRUE) -> ("count out"=→"Sends 2":u32)  [unwired: 14 in]
      }
    }
    n187 = Bundle By Name(cluster=w58, "EnableFIFO"=w56) -> (w57:T7)
    n188 = Bundle By Name(cluster=T7 {"EnableFIFO"=FALSE, "EnableStages"={"FreqShiftEnable"=FALSE, "Step4Enable"=FALSE, "Step5Enable"=FALSE, "Step6Enable"=FALSE, "Step7Enable"=FALSE}}, "EnableFIFO"=w51, "EnableStages"="Enable 2") -> (w43:T7)
    n189 = feedback #64() -> (w126:fxp<+/-,48,0>)  [unwired: 1 in]
    n190 = feedback-in #64("FreqShiftCal 2") -> ()
    n191 = feedback #65() -> (w118:T2)  [unwired: 1 in]
    n192 = feedback-in #65("Scale 2") -> ()
    n193 = feedback #66() -> (w124:fxp<+/-,48,0>)  [unwired: 1 in]
    n194 = feedback-in #66("FreqShiftBeac 2") -> ()
    n195 = Bundle By Name(cluster=w43, "EnableFIFO"=w45) -> (w44:T7)
    n196 = call "20210319_Shift_00_ATA_FPGA.vi"("Scale"=w132, "Input valid"=w147, "Index"=w17, "Enable"=w58, "frequency shift"=w128, "Data in"=w211) -> ("Q Shift Output"=w146:T9, "I Shift Output"=w140:T9)  [unwired: 4 in]
    n197 = call "20210319_Shift_00_ATA_FPGA.vi"("Scale"=w118, "Input valid"=w141, "Index"=w17, "Enable"=w43, "frequency shift"=w126, "Data in"=w210) -> ("Q Shift Output"=w42:T9, "I Shift Output"=w50:T9)  [unwired: 4 in]
    n198 = call "20210319_Shift_00_ATA_FPGA.vi"("Scale"=w132, "Input valid"=w147, "Index"=w17, "Enable"=w57, "frequency shift"=w130, "Data in"=w211) -> ("Q Shift Output"=w225:T9, "I Shift Output"=w137:T9)  [unwired: 4 in]
    n199 = call "20210319_Shift_00_ATA_FPGA.vi"("Scale"=w118, "Input valid"=w141, "Index"=w17, "Enable"=w44, "frequency shift"=w124, "Data in"=w210) -> ("Q Shift Output"=w31:T9, "I Shift Output"=w35:T9)  [unwired: 4 in]
    n200 = Unbundle By Name(w140) -> ("output valid"=w72:bool, "Data out"=w65:fxp<+/-,24,1>, "Index"=w67:fxp<+/-,24,1>, "Probe"=w74:T1)
    n201 = Unbundle By Name(w146) -> ("Data out"=w63:fxp<+/-,24,1>, "Index"=w73:fxp<+/-,24,1>, "Probe"=w53:T1)
    n202 = Unbundle By Name(w225) -> ("Data out"=w70:fxp<+/-,24,1>, "Index"=w25:fxp<+/-,24,1>, "Probe"=w69:T1)
    "AI0_Co_Beac_Q_Index" <- w25
    n203 = Unbundle By Name(w50) -> ("output valid"=w49:bool, "Data out"=w48:fxp<+/-,24,1>, "Index"=w47:fxp<+/-,24,1>, "Probe"=w41:T1)
    n204 = Unbundle By Name(w42) -> ("Data out"=w38:fxp<+/-,24,1>, "Index"=w37:fxp<+/-,24,1>, "Probe"=w40:T1)
    n205 = Unbundle By Name(w137) -> ("Probe"=w71:T1, "Data out"=w68:fxp<+/-,24,1>, "Index"=w55:fxp<+/-,24,1>)
    "AI0_Co_I_Index" <- w55
    n206 = Unbundle By Name(w35) -> ("Data out"=w32:fxp<+/-,24,1>, "Index"=w33:fxp<+/-,24,1>, "Probe"=w34:T1)
    n207 = Unbundle By Name(w31) -> ("Data out"=w29:fxp<+/-,24,1>, "Index"=w27:fxp<+/-,24,1>, "Probe"=w30:T1)
    n208 = feedback #67() -> (→"AI0_Cal_IProbe":T1)  [unwired: 1 in]
    n209 = feedback-in #67(w74) -> ()
    n210 = feedback #68() -> (→"Chan0_Cal_QProbe":T1)  [unwired: 1 in]
    n211 = feedback-in #68(w53) -> ()
    n212 = feedback #69() -> (→"Chan0_Beac_IProbe":T1)  [unwired: 1 in]
    n213 = feedback-in #69(w71) -> ()
    n214 = feedback #70() -> (→"Chan0_Beac_QProbe":T1)  [unwired: 1 in]
    n215 = feedback-in #70(w69) -> ()
    n216 = feedback #71() -> (→"Chan1_Cal_IProbe":T1)  [unwired: 1 in]
    n217 = feedback-in #71(w41) -> ()
    n218 = feedback #72() -> (→"Chan1_Cal_QProbe":T1)  [unwired: 1 in]
    n219 = feedback-in #72(w40) -> ()
    n220 = feedback #73() -> (→"Chan1_Beac_IProbe":T1)  [unwired: 1 in]
    n221 = feedback-in #73(w34) -> ()
    n222 = feedback #74() -> (→"Chan1_Beac_QProbe":T1)  [unwired: 1 in]
    n223 = feedback-in #74(w30) -> ()
    n224 = And(x=w72, y="EnableFIFO") -> (x .and. y?=w16:bool)
    "Write to FIFO" <- w16
    n225 = And(x="EnableFIFO", y=w49) -> (x .and. y?=w15:bool)
    n226 = case shown="True" w227 {
      tunnel: w221 -> [_ w301]
      frame False {
      }
      frame True {
        n227 = xnode "VI-Defined FIFO Configuration"() -> ("FIFO Out"=w296:refnum<k21>)
        n228 = xnode ("FIFO Method Node")("Element"=w301, "Timeout"=0, "FIFO In"=w296) -> ("Timed Out?"=→"NoiseFloorFIFOTimeOut":bool)  [unwired: 1 out]
        n229 = call-poly <instrlib>:"Count Up.vi"("increment"=TRUE) -> ("count out"=→"Sends":u32)  [unwired: 14 in]
      }
    }
    n230 = feedback #75() -> (w222:bool)  [unwired: 1 in]
    n231 = feedback-in #75(w16) -> ()
    n232 = feedback #76() -> (w223:fxp<+/-,24,1>)  [unwired: 1 in]
    n233 = feedback-in #76(w65) -> ()
    n234 = feedback #77() -> (w66:fxp<+/-,24,1>)  [unwired: 1 in]
    n235 = feedback-in #77(w67) -> ()
    n236 = feedback #78() -> (w62:fxp<+/-,24,1>)  [unwired: 1 in]
    n237 = feedback-in #78(w63) -> ()
    n238 = feedback #79() -> (w144:fxp<+/-,24,1>)  [unwired: 1 in]
    n239 = feedback-in #79(w73) -> ()
    n240 = feedback #80() -> (w145:fxp<+/-,24,1>)  [unwired: 1 in]
    n241 = feedback-in #80(w68) -> ()
    n242 = feedback #81() -> (w54:fxp<+/-,24,1>)  [unwired: 1 in]
    n243 = feedback-in #81(w55) -> ()
    n244 = feedback #82() -> (w224:fxp<+/-,24,1>)  [unwired: 1 in]
    n245 = feedback-in #82(w70) -> ()
    n246 = feedback #83() -> (w64:fxp<+/-,24,1>)  [unwired: 1 in]
    n247 = feedback-in #83(w25) -> ()
    n248 = feedback #84() -> (w13:bool)  [unwired: 1 in]
    "Write to FIFO 2" <- w13
    n249 = feedback-in #84(w15) -> ()
    n250 = feedback #85() -> (w197:fxp<+/-,24,1>)  [unwired: 1 in]
    n251 = feedback-in #85(w48) -> ()
    n252 = feedback #86() -> (w39:fxp<+/-,24,1>)  [unwired: 1 in]
    n253 = feedback-in #86(w47) -> ()
    n254 = feedback #87() -> (w142:fxp<+/-,24,1>)  [unwired: 1 in]
    n255 = feedback-in #87(w38) -> ()
    n256 = feedback #88() -> (w36:fxp<+/-,24,1>)  [unwired: 1 in]
    n257 = feedback-in #88(w37) -> ()
    n258 = feedback #89() -> (w143:fxp<+/-,24,1>)  [unwired: 1 in]
    n259 = feedback-in #89(w32) -> ()
    n260 = feedback #90() -> (w196:fxp<+/-,24,1>)  [unwired: 1 in]
    n261 = feedback-in #90(w33) -> ()
    n262 = feedback #91() -> (w28:fxp<+/-,24,1>)  [unwired: 1 in]
    n263 = feedback-in #91(w29) -> ()
    n264 = feedback #92() -> (w26:fxp<+/-,24,1>)  [unwired: 1 in]
    n265 = feedback-in #92(w27) -> ()
    n266 = case shown="True" w222 {
      tunnel: w223 -> [_ w315]
      tunnel: w224 -> [_ w304]
      tunnel: w145 -> [_ w302]
      tunnel: w144 -> [_ w310]
      tunnel: w66 -> [_ w313]
      tunnel: w62 -> [_ w311]
      tunnel: w64 -> [_ w312]
      tunnel: w54 -> [_ w309]
      frame False {
        # "Ready last time?"
      }
      frame True {
        # "Ramp function can be enabled\nfor test/debug"
        # "Transfer when data is valid.\nMost of the time the data is NOT\nvalid as a result of drastic decimation"
        n267 = call-poly <instrlib>:"Count Up.vi"("increment"=TRUE) -> ("count out"=w317:u32)  [unwired: 14 in]
        n268 = To Fixed-Point(fixed-point type=fxp<+/-,24,1> 0.0, number=w317) -> (fixed-point=w316:fxp<+/-,24,1>)
        n269 = feedback-in #93(w316) -> ()
        n270 = feedback #93() -> (w306:fxp<+/-,24,1>)  [unwired: 1 in]
        n271 = Select(t=w306, s="Ramp?", f=w315) -> (s? t:f=w314:fxp<+/-,24,1>)
        n272 = Select(t=w306, s="Ramp?", f=w302) -> (s? t:f=w303:fxp<+/-,24,1>)
        n273 = Build Array(w314, w313, w311, w310, w303, w309, w304, w312) -> (w308:fxp<+/-,24,1>[])
        n274 = xnode ("FIFO Method Node")("Element"=w308, "Timeout"=0) -> ()  [unwired: 1 in, 2 out]
      }
    }
    n275 = case shown="True" w13 {
      tunnel: w197 -> [_ w294]
      tunnel: w196 -> [_ w290]
      tunnel: w143 -> [_ w282]
      tunnel: w142 -> [_ w292]
      tunnel: w39 -> [_ w293]
      tunnel: w36 -> [_ w291]
      tunnel: w28 -> [_ w289]
      tunnel: w26 -> [_ w288]
      frame False {
      }
      frame True {
        # "Ramp function can be enabled\nfor test/debug"
        # "Transfer when data is valid.\nMost of the time the data is NOT\nvalid as a result of drastic decimation"
        n276 = call-poly <instrlib>:"Count Up.vi"("increment"=TRUE) -> ("count out"=w285:u32)  [unwired: 14 in]
        n277 = To Fixed-Point(fixed-point type=fxp<+/-,24,1> 0.0, number=w285) -> (fixed-point=w284:fxp<+/-,24,1>)
        n278 = local read "Ramp?"() -> (w280:bool)
        n279 = feedback #94() -> (w283:fxp<+/-,24,1>)  [unwired: 1 in]
        n280 = feedback-in #94(w284) -> ()
        n281 = Select(t=w283, s=w280, f=w282) -> (s? t:f=w281:fxp<+/-,24,1>)
        n282 = Build Array(w294, w293, w292, w291, w281, w290, w289, w288) -> (w295:fxp<+/-,24,1>[])
        n283 = xnode ("FIFO Method Node")("Element"=w295, "Timeout"=0) -> ()  [unwired: 1 in, 2 out]
      }
    }
  }
  n284 = while {
    stop <- FALSE stop-if-true
    # "Initialization Done:\nThis node will be true when the Adapter Module has finished configuring itself and is generating valid samples."
    # "Configuration Loop"
    n285 = xnode "FPGA I/O Node"() -> ("IO Module\\Initialization Done"=→"IO Module\\Initialization Done")  [unwired: 1 in, 1 out]
  }
  n286 = while {
    stop <- FALSE stop-if-true
    # "Clock Commit has a built in rising edge detector. Refer to the NI 5762 Component-Level IP Reference section of the LabVIEW FPGA Module Help for more information."
    # "This loop configures the Sample clock selection for the NI 5762. Refer to the Clock Select (Host).vi Host VI for more information about how this example configures the clock."
    n287 = xnode "FPGA I/O Node"("IO Module\\Sample Clock Select"="Sample Clock Select", "IO Module\\Sample Clock Commit"="Sample Clock Commit") -> ("IO Module\\SPI Idle"=→"SPI Idle", "IO Module\\Configuration Error"=→"Configuration Error", "IO Module\\PLL Locked"=→"Synthesizer Locked")  [unwired: 5 in, 5 out]
  }
  n288 = xnode "VI-Defined Memory"() -> ("Memory Out"=w6:refnum<k21>)
  n289 = xnode "VI-Defined Memory"() -> ("Memory Out"=w5:refnum<k21>)
  n290 = for {
    N: 8192 ("dimension size") -> [_]
    tunnel: [w331] -> w7
    tunnel: w6 -> [w330]
    i -> [w334]
    n291 = To Unsigned Long Integer(number=w334) -> (unsigned 32bit integer=w333:u32)
    n292 = xnode ("Memory Method Node")("Address"=w333, "Data"=fxp<+/-,27,12> 0.0, "Memory In"=w330) -> ("Memory Out"=w331:refnum<k21>)
  }
  n293 = for {
    N: 8192 ("dimension size") -> [_]
    tunnel: [w336] -> w4
    tunnel: w5 -> [w335]
    i -> [w339]
    n294 = To Unsigned Long Integer(number=w339) -> (unsigned 32bit integer=w338:u32)
    n295 = xnode ("Memory Method Node")("Address"=w338, "Data"=fxp<+/-,27,12> 0.0, "Memory In"=w335) -> ("Memory Out"=w336:refnum<k21>)
  }
  n296 = while {
    shift-right: [w342] -> _
    shift-left: TRUE -> [w343]
    tunnel: w7 -> [w340]
    i -> [w344]
    stop <- FALSE stop-if-true
    # "Most recent processed point"
    # "Noise Floor FFT"
    n297 = xnode ("FIFO Method Node")("Timeout"=0) -> ("Element"=w346:fxp<+/-,16,1>, "Timed Out?"=w341:bool)  [unwired: 1 in, 1 out]
    "ReceiverTimed Out" <- w341
    n298 = case shown="False" w341 {
      tunnel: w346 -> [w373 _]
      tunnel: w343 -> [w372 w405]
      tunnel: [FALSE w405] -> w342
      tunnel: w340 -> [w354 _]
      frame False {
        # "Squaring FFT values so we can add them. \nOtherwise we get destructive interference and the averaging doesn't work."
        # "Must be greater/equal.\nEqual can get stuck if the user\ndecreases #Avg value.\n3-14-2019"
        # "Is collection of frames finished?"
        # "Is frame finished?"
        # "Build sum of many FFT frames, point by point."
        n299 = xnode ("FFT")("real data in"=w373, "reset"=w372, "imaginary data in"=fxp<+/-,16,1> 0.0) -> ("data index"=w365:u16, "real data out"=w351:fxp<+/-,30,15>)  [unwired: 1 out]
        n300 = To Unsigned Long Integer(number=w365) -> (unsigned 32bit integer=w357:u32)
        n301 = xnode ("Memory Method Node")("Address"=w357, "Memory In"=w354) -> ("Data"=w356:fxp<+/-,27,12>, "Memory Out"=w353:refnum<k21>)
        n302 = feedback #95() -> (w367:u16)  [unwired: 1 in]
        n303 = feedback-in #95(w365) -> ()
        n304 = xnode ("High Throughput Multiply")("x"=w351, "y"=w351) -> ("x*y"=w350:fxp<+/-,60,30>)
        n305 = Build Array(w365, w367) -> (→"SuccessiveIndeces":u16[])
        n306 = To Fixed-Point(fixed-point type=fxp<+/-,27,12> 0.0 ("Data"), number=w350) -> (fixed-point=w348:fxp<+/-,27,12>)
        n307 = xnode ("High Throughput Add")("x"=w356, "y"=w348) -> ("x+y"=w355:fxp<+/-,28,13>)  [unwired: 1 out]
        n308 = To Fixed-Point(fixed-point type=fxp<+/-,27,12> 0.0 ("Data"), number=w355) -> (fixed-point=w358:fxp<+/-,27,12>)
        n309 = Greater Or Equal?(x=w365, y=u16 8191) -> (x >= y?=w360:bool)
        n310 = xnode ("Memory Method Node")("Address"=w357, "Data"=w358, "Memory In"=w353) -> ("Memory Out"=w352:refnum<k21>)
        n311 = feedback #96(FALSE) -> (w363:bool)
        n312 = call-poly <instrlib>:"Count Up.vi"("increment"=w360, "reset"=w363) -> ("count out"=w362:u16)  [unwired: 13 in]
        n313 = Greater Or Equal?(x=w362, y="#Avg") -> (x >= y?=w370:bool)
        n314 = feedback-in #96(w370) -> ()
        n315 = case shown="True" w370 {
          tunnel: w352 -> [_ w393]
          frame False {
          }
          frame True {
            n316 = for {
              N: 8192 ("dimension size") -> [_]
              tunnel: w393 -> [w395]
              i -> [w398]
              # "Transfer summed collection of frames to host."
              # "Reset to zeros"
              n317 = To Unsigned Long Integer(number=w398) -> (unsigned 32bit integer=w400:u32)
              n318 = xnode ("Memory Method Node")("Address"=w400, "Memory In"=w395) -> ("Data"=w399:fxp<+/-,27,12>, "Memory Out"=w396:refnum<k21>)
              n319 = Integer to Fixed-Point Cast(fixed-point type=fxp<+/-,30,15> 0.0 ("real data out"), integer=w398) -> (fixed-point=w403:fxp<+/-,30,15>)
              n320 = Build Array(w403, w399) -> (w401:fxp<+/-,30,15>[])
              n321 = xnode ("Memory Method Node")("Address"=w400, "Data"=fxp<+/-,27,12> 0.0, "Memory In"=w396) -> ()  [unwired: 1 out]
              n322 = xnode ("FIFO Method Node")("Element"=w401, "Timeout"=0) -> ()  [unwired: 1 in, 2 out]
            }
          }
        }
      }
      frame True {
      }
    }
    "NoiseFloorFFT_LoopCount" <- w344
  }
  n323 = while {
    shift-right: [w408] -> _
    shift-left: TRUE -> [w409]
    tunnel: w4 -> [w406]
    i -> [w410]
    stop <- FALSE stop-if-true
    # "Most recent processed point"
    # "Noise Floor FFT"
    n324 = xnode ("FIFO Method Node")("Timeout"=0) -> ("Element"=w412:fxp<+/-,16,1>, "Timed Out?"=w407:bool)  [unwired: 1 in, 1 out]
    "ReceiverTimed Out 2" <- w407
    n325 = case shown="False" w407 {
      tunnel: w412 -> [w439 _]
      tunnel: w409 -> [w438 w471]
      tunnel: [FALSE w471] -> w408
      tunnel: w406 -> [w420 _]
      frame False {
        # "Is collection of frames finished?"
        # "Is frame finished?"
        # "Build sum of many FFT frames, point by point."
        n326 = xnode ("FFT 2")("real data in"=w439, "reset"=w438, "imaginary data in"=fxp<+/-,16,1> 0.0) -> ("data index"=w431:u16, "real data out"=w415:fxp<+/-,30,15>)  [unwired: 1 out]
        n327 = To Unsigned Long Integer(number=w431) -> (unsigned 32bit integer=w423:u32)
        n328 = xnode ("Memory Method Node")("Address"=w423, "Memory In"=w420) -> ("Data"=w422:fxp<+/-,27,12>, "Memory Out"=w419:refnum<k21>)
        n329 = feedback #97() -> (w433:u16)  [unwired: 1 in]
        n330 = feedback-in #97(w431) -> ()
        n331 = xnode ("High Throughput Multiply")("x"=w415, "y"=w415) -> ("x*y"=w417:fxp<+/-,60,30>)
        n332 = Build Array(w431, w433) -> (→"SuccessiveIndeces 2":u16[])
        n333 = To Fixed-Point(fixed-point type=fxp<+/-,27,12> 0.0 ("Data"), number=w417) -> (fixed-point=w414:fxp<+/-,27,12>)
        n334 = xnode ("High Throughput Add")("x"=w422, "y"=w414) -> ("x+y"=w421:fxp<+/-,28,13>)  [unwired: 1 out]
        n335 = To Fixed-Point(fixed-point type=fxp<+/-,27,12> 0.0 ("Data"), number=w421) -> (fixed-point=w424:fxp<+/-,27,12>)
        n336 = Greater Or Equal?(x=w431, y=u16 8191) -> (x >= y?=w426:bool)
        n337 = xnode ("Memory Method Node")("Address"=w423, "Data"=w424, "Memory In"=w419) -> ("Memory Out"=w418:refnum<k21>)
        n338 = feedback #98(FALSE) -> (w429:bool)
        n339 = call-poly <instrlib>:"Count Up.vi"("increment"=w426, "reset"=w429) -> ("count out"=w428:u16)  [unwired: 13 in]
        n340 = Greater Or Equal?(x=w428, y="#Avg 2") -> (x >= y?=w436:bool)
        n341 = feedback-in #98(w436) -> ()
        n342 = case shown="True" w436 {
          tunnel: w418 -> [_ w459]
          frame False {
          }
          frame True {
            n343 = for {
              N: 8192 ("dimension size") -> [_]
              tunnel: w459 -> [w461]
              i -> [w464]
              # "Transfer summed collection of frames to host."
              # "Reset to zeros"
              n344 = To Unsigned Long Integer(number=w464) -> (unsigned 32bit integer=w466:u32)
              n345 = xnode ("Memory Method Node")("Address"=w466, "Memory In"=w461) -> ("Data"=w465:fxp<+/-,27,12>, "Memory Out"=w462:refnum<k21>)
              n346 = Integer to Fixed-Point Cast(fixed-point type=fxp<+/-,30,15> 0.0 ("real data out"), integer=w464) -> (fixed-point=w469:fxp<+/-,30,15>)
              n347 = Build Array(w469, w465) -> (w467:fxp<+/-,30,15>[])
              n348 = xnode ("Memory Method Node")("Address"=w466, "Data"=fxp<+/-,27,12> 0.0, "Memory In"=w462) -> ()  [unwired: 1 out]
              n349 = xnode ("FIFO Method Node")("Element"=w467, "Timeout"=0) -> ()  [unwired: 1 in, 2 out]
            }
          }
        }
      }
      frame True {
      }
    }
    "NoiseFloorFFT_LoopCount 2" <- w410
  }
  n350 = node-c288(w11) -> ()
